vi "121.vi"(10 "V' x A":dbl[](array[numeric]), 11 "Array in":dbl[](array[numeric])) -> (2 "interleaved array":dbl[](array[numeric]))   [LabVIEW 2017]
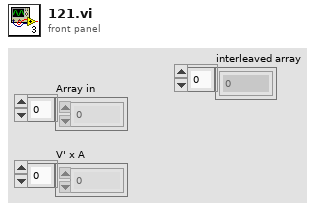
[diagram p1: front panel]
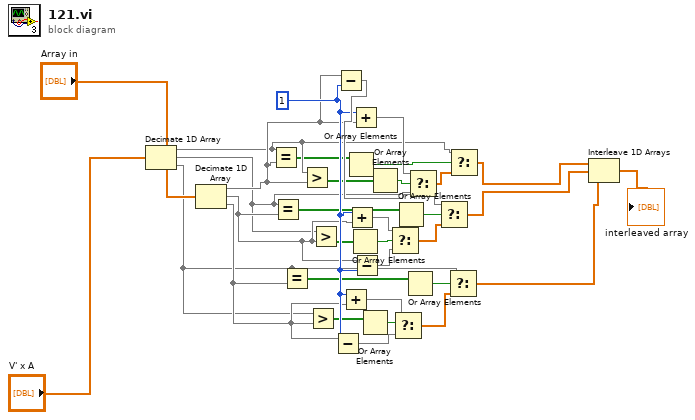
[diagram p0: block diagram]
diagram:
  w33 = 1
  n1 = Decimate 1D Array("V' x A") -> (w30:dbl[], w22:dbl[], w17:dbl[])
  n2 = Decimate 1D Array("Array in") -> (w32:dbl[], w26:dbl[], w21:dbl[])
  n3 = Equal?(x=w30, y=w32) -> (x = y?=w11:bool[])
  n4 = Equal?(x=w22, y=w26) -> (x = y?=w8:bool[])
  n5 = Equal?(x=w17, y=w21) -> (x = y?=w7:bool[])
  n6 = Greater?(x=w30, y=w32) -> (0:w29:bool[])
  n7 = Greater?(x=w17, y=w21) -> (0:w16:bool[])
  n8 = Greater?(x=w22, y=w26) -> (0:w23:bool[])
  n9 = Subtract(x=w21, y=w33) -> (x-y=w20:dbl[])
  n10 = Subtract(x=w32, y=w33) -> (x-y=w34:dbl[])
  n11 = Add(x=w33, y=w21) -> (x+y=w19:dbl[])
  n12 = Or Array Elements(Boolean array=w11) -> (logical OR=w10:bool)
  n13 = Add(x=w33, y=w26) -> (x+y=w25:dbl[])
  n14 = Or Array Elements(Boolean array=w23) -> (logical OR=w24:bool)
  n15 = Add(x=w33, y=w32) -> (x+y=w31:dbl[])
  n16 = Subtract(x=w26, y=w33) -> (x-y=w1:dbl[])
  n17 = Or Array Elements(Boolean array=w16) -> (logical OR=w15:bool)
  n18 = Or Array Elements(Boolean array=w29) -> (logical OR=w28:bool)
  n19 = Select(t=w25, s=w24, f=w1) -> (s? t:f=w13:dbl[])
  n20 = Select(t=w19, s=w15, f=w20) -> (s? t:f=w14:dbl[])
  n21 = Or Array Elements(Boolean array=w8) -> (logical OR=w9:bool)
  n22 = Or Array Elements(Boolean array=w7) -> (logical OR=w6:bool)
  n23 = Select(t=w31, s=w28, f=w34) -> (s? t:f=w27:dbl[])
  n24 = Select(t=w22, s=w9, f=w13) -> (s? t:f=w4:dbl[])
  n25 = Select(t=w17, s=w6, f=w14) -> (s? t:f=w3:dbl[])
  n26 = Select(t=w30, s=w10, f=w27) -> (s? t:f=w5:dbl[])
  n27 = Interleave 1D Arrays(w5, w4, w3) -> (→"interleaved array":dbl[])
